vi "Revision Query.vi"(8 "error in (no error)":errorcluster, 11 "VISA resource name":refnum<visa-resource-name>) -> (0 "error out":errorcluster, 1 "Firmware Revision":string, 2 "Instrument Driver Revision":string, 3 "VISA resource name out":refnum<visa-resource-name>, 5 "Instrument Identification":string)   [LabVIEW 2015, in "Rohde&Schwarz CMXP NR FR2 Measurement.lvlib"]
doc: "This VI returns the revision numbers of the instrument driver and instrument firmware.\n\nAttribute:\n-\n\nRemote-control command:\n*IDN?"
uses:
  <instrlib>/Rohde&Schwarz CMXP NR FR2 Measurement/Rohde&Schwarz CMXP NR FR2 Measurement.lvlib
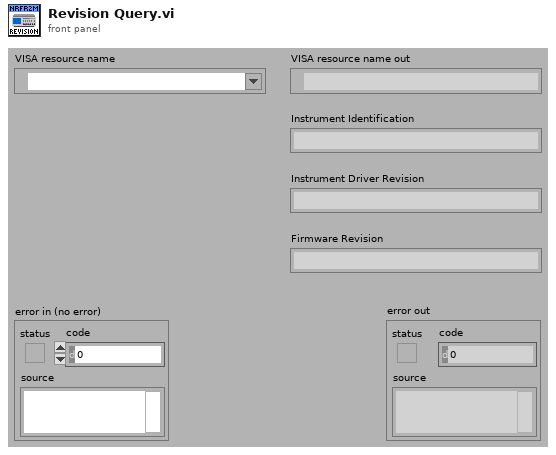
[diagram p1: front panel]
types:
  T1 = cluster{"Major":u16, "Minor":u16, "Fix":u16, "Build":u16}
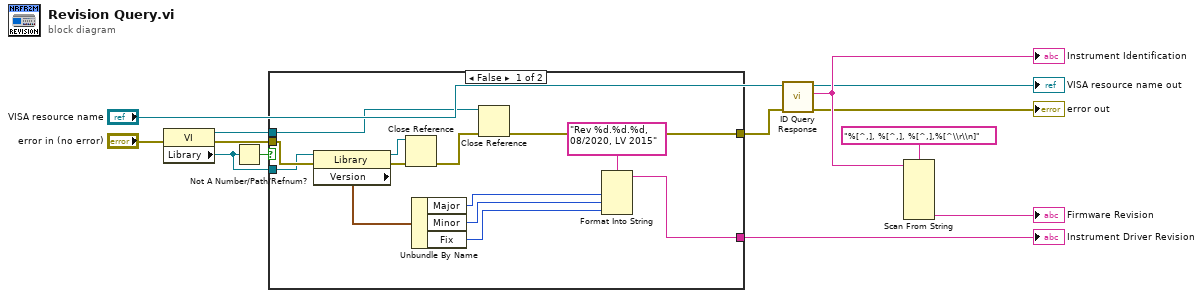
[diagram p0: block diagram]
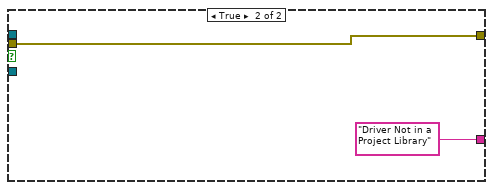
[diagram p2: hidden frame]
diagram:
  n1 = property on="Property Node" class="VI"(error in="error in (no error)") -> (reference out=w11:refnum<vi>, error out=w10:errorcluster, "Library"=w9:refnum<vi>)  [unwired: 1 in]
  n2 = Not A Number/Path/Refnum?(number/path/refnum=w9) -> (NaN/Path/Refnum?=w8:bool)
  n3 = case shown="False" w8 {
    tunnel: w11 -> [w23 _]
    tunnel: w10 -> [w21 w28]
    tunnel: [w20 w28] -> w3
    tunnel: [w18 "Driver Not in a Project Library"] -> w7
    tunnel: w9 -> [w19 _]
    frame False {
      n4 = property on="Property Node" class="Library"(reference=w19, error in=w21) -> (reference out=w25:refnum<vi>, error out=w26:errorcluster, "Version"=w17:T1)
      n5 = Close Reference(reference=w25, error in (no error)=w26) -> (error out=w24:errorcluster)
      n6 = Unbundle By Name(w17) -> ("Major"=w16:u16, "Minor"=w15:u16, "Fix"=w14:u16)
      n7 = Close Reference(reference=w23, error in (no error)=w24) -> (error out=w20:errorcluster)
      n8 = Format Into String(format string="Rev %d.%d.%d, 08/2020, LV 2015", w16, w15, w14) -> (resulting string=w18:string)  [unwired: 2 in, 1 out]
    }
    frame True {
    }
  }
  "Instrument Driver Revision" <- w7
  n9 = call <instrlib>:"ID Query Response.vi"("error in (no error)"=w3, "VISA resource name"="VISA resource name") -> ("error out"=→"error out":errorcluster, "ID Query Response"=w5:string, "VISA resource name out"=→"VISA resource name out":refnum<visa-resource-name>)  [unwired: 7 in]
  "Instrument Identification" <- w5
  n10 = Scan From String(format string="%[^,], %[^,], %[^,],%[^\\r\\n]", input string=w5) -> (output 4=→"Firmware Revision":string)  [unwired: 9 in, 3 out]
